vi "ToExcelTemplate.vi"(7 "Repport Type":enum16{"Weekly SR Data", "SR Trends"}(ring), 8 "error in (no error)":errorcluster, 10 "Data In":string[][](array[string])=[[" ", "Week 1", "Week 2", "Week 3", "Week 4", "Week 5", "Week 6", "Week 7", "Week 8", "Week 9", "Week 10", "Week 11", "Week 12", "Week 13", "Week 14", "Week 15", "Week 16", "Week 17", "Week 18"], ["AE-Poland", "5", "17", "13", "8", "20", "22", "20", "25", "17", "21", "14", "13", "13", "18", "10", "7", "5", "5"], ["AE-Czech and Slovakia", "19", "26", "22", "16", "21", "18", "20", "19", "28", "23", "29", "17", "20", "23", "22", "15", "19", "15"], ["AE-Hungary", "7", "11", "5", "10", "8", "14", "4", "13", "15", "6", "13", "6", "14", "4", "7", "13", "9", "3"], ["AE-Romania", "5", "11", "11", "8", "9", "9", "10", "9", "9", "11", "17", "12", "9", "7", "7", "12", "5", "1"]]) -> (0 "error out":errorcluster, 2 "Data Out":string[][](array[string])=[[" ", "Week 1", "Week 2", "Week 3", "Week 4", "Week 5", "Week 6", "Week 7", "Week 8", "Week 9", "Week 10", "Week 11", "Week 12", "Week 13", "Week 14", "Week 15", "Week 16", "Week 17", "Week 18"], ["AE-Poland", "5", "17", "13", "8", "20", "22", "20", "25", "17", "21", "14", "13", "13", "18", "10", "7", "5", "5"], ["AE-Czech and Slovakia", "19", "26", "22", "16", "21", "18", "20", "19", "28", "23", "29", "17", "20", "23", "22", "15", "19", "15"], ["AE-Hungary", "7", "11", "5", "10", "8", "14", "4", "13", "15", "6", "13", "6", "14", "4", "7", "13", "9", "3"], ["AE-Romania", "5", "11", "11", "8", "9", "9", "10", "9", "9", "11", "17", "12", "9", "7", "7", "12", "5", "1"]], 3 "TemplatePath Out":path)   [LabVIEW 2017, in "DS_Lib.lvlib" / "SRReportParser.lvlib"]
uses:
  SRReportParser.lvlib
  <vilib>/addons/_office/excel.llb/Excel Easy Table (str).vi
  <vilib>/Utility/NIReport.llb/NI_report.lvclass
  <vilib>/addons/_office/NI_ReportGenerationToolkit.lvlib
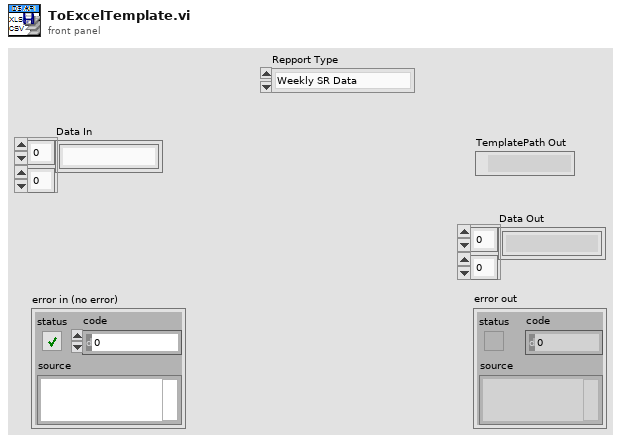
[diagram p1: front panel]
types:
  T1 = enum16{"maximized", "minimized", "normal", "no change"}
  T2 = enum16{"Standard Report", "HTML", "Word", "Excel"}
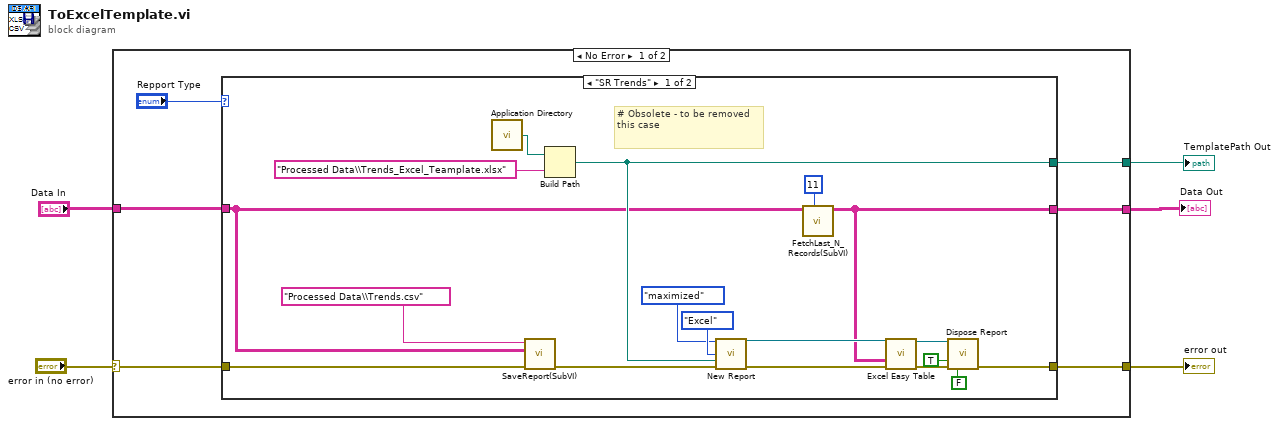
[diagram p0: block diagram]
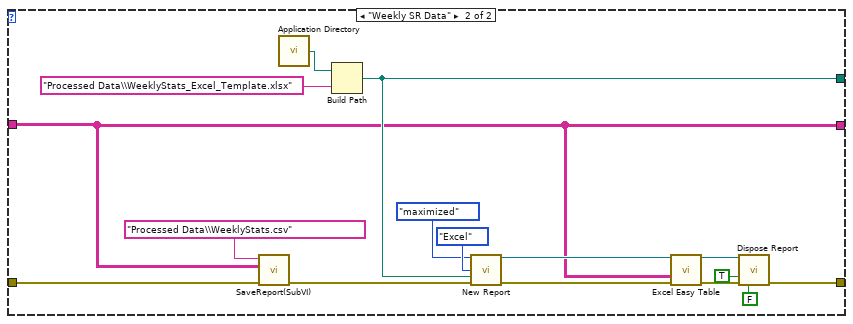
[diagram p2: hidden frame]
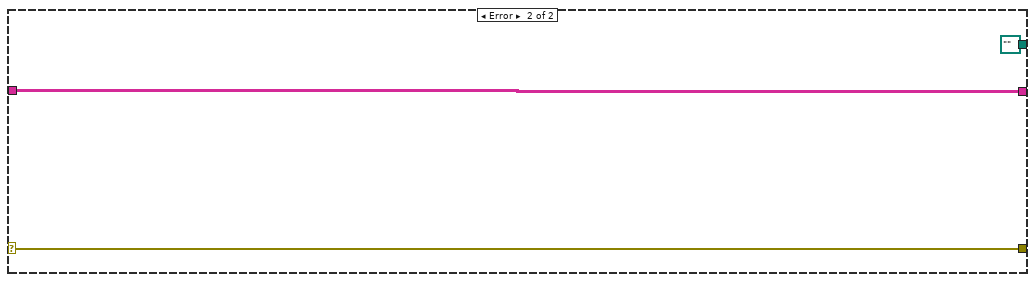
[diagram p3: hidden frame]
diagram:
  n1 = case shown="No Error" "error in (no error)" {
    selector: "error in (no error)" -> [w9 w47]
    tunnel: [w11 path "" ("appended path")] -> w5
    tunnel: [w10 w47] -> w4
    tunnel: "Data In" -> [w7 w48]
    tunnel: [w6 w48] -> w1
    frame No Error {
      n2 = case shown="\"SR Trends\"" "Repport Type" {
        tunnel: [w23 w37] -> w11
        tunnel: [w20 w34] -> w10
        tunnel: w9 -> [w19 w32]
        tunnel: w7 -> [w14 w30]
        tunnel: [w12 w30] -> w6
        frame "SR Trends" {
          # "# Obsolete - to be removed this case"
          n3 = call <vilib>:"Application Directory.vi"() -> ("Application Directory"=w28:path)
          n4 = call "SaveReport(SubVI).vi"("Error In"=w19, "2D Data"=w14, "FileName"="Processed Data\\Trends.csv" ("name or relative path")) -> ("Error Out"=w18:errorcluster)  [unwired: 8 in]
          n5 = Build Path(base path=w28, name or relative path="Processed Data\\Trends_Excel_Teamplate.xlsx") -> (appended path=w23:path)
          n6 = call <vilib>:"New Report.vi"("window state (normal)"=T1."maximized", "report type"=T2."Excel", "template (empty)"=w23, "error in (no error)"=w18) -> ("report out"=w15:refnum<class "NI_report.lvclass">, "error out"=w16:errorcluster)  [unwired: 10 in]
          n7 = call "FetchLast_N_Records(SubVI).vi"("# of Records"=11, "Data In in"=w14) -> ("Data In out"=w12:string[][])  [unwired: 9 in]
          n8 = call-poly <vilib>:"Excel Easy Table.vi"("report in"=w15, "text data"=w12, "error in (no error)"=w16) -> ("report out"=w24:refnum<class "NI_report.lvclass">, "error out"=w25:errorcluster)  [unwired: 8 in, 3 out]
          n9 = call-dynamic "Dispose Report.vi"("report in"=w24, "save changes? (F)"=TRUE, "error in (no error)"=w25, "close report? (T)"=FALSE) -> ("error out"=w20:errorcluster)  [unwired: 11 in]
        }
        frame "Weekly SR Data" {
          n10 = call "SaveReport(SubVI).vi"("Error In"=w32, "2D Data"=w30, "FileName"="Processed Data\\WeeklyStats.csv" ("name or relative path")) -> ("Error Out"=w31:errorcluster)  [unwired: 8 in]
          n11 = call <vilib>:"Application Directory.vi"() -> ("Application Directory"=w44:path)
          n12 = Build Path(base path=w44, name or relative path="Processed Data\\WeeklyStats_Excel_Template.xlsx") -> (appended path=w37:path)
          n13 = call <vilib>:"New Report.vi"("window state (normal)"=T1."maximized", "report type"=T2."Excel", "template (empty)"=w37, "error in (no error)"=w31) -> ("report out"=w42:refnum<class "NI_report.lvclass">, "error out"=w41:errorcluster)  [unwired: 10 in]
          n14 = call-poly <vilib>:"Excel Easy Table.vi"("report in"=w42, "text data"=w30, "error in (no error)"=w41) -> ("report out"=w38:refnum<class "NI_report.lvclass">, "error out"=w39:errorcluster)  [unwired: 8 in, 3 out]
          n15 = call-dynamic "Dispose Report.vi"("report in"=w38, "save changes? (F)"=TRUE, "error in (no error)"=w39, "close report? (T)"=FALSE) -> ("error out"=w34:errorcluster)  [unwired: 11 in]
        }
      }
    }
    frame Error {
    }
  }
  "TemplatePath Out" <- w5
  "error out" <- w4
  "Data Out" <- w1
